vi "ADIS16448 IMU Example.vi"() -> ()   [LabVIEW 2019]
uses:
  <vilib>/Utility/RT CPU Load.ctl
  ADIS16448Lib/Typedef/ADIS16448 Hardware Configuration.ctl
  <vilib>/Rock Robotics/WPI/SPI/WPI_SPIMode.ctl
  <vilib>/Rock Robotics/SystemInterfaces/DIO/FPGA_DIOChannel.ctl
  <vilib>/Rock Robotics/SystemInterfaces/spilib/spi_bus.ctl
  <vilib>/NI_Real-Time Target Support.lvlib
panel:
  in  "Initial Calibration Time (sec)":i32=5
  in  "Hardware Config":T1={"SPI Clock Rate (Hz)"=1000000.0, "IMU SPI Mode (3)"=enum."Mode 3 (Clk Idle High,Sample on Trailing)", "IMU Reset Pin"=enum."DIO MXP 8", "IMU SPI Bus"=enum."SPI MXP", "IMU Data Ready Pin"=enum."DIO MXP 0", "Stall Config"={"Pow2BytesPerRead"=1, "StallTicks"=1000, "CsToSclkTicks"=5}, "IMU Status LED Pin"=enum."DIO MXP 9"}
  in  "Recalibrate?":bool
  in  "Reset?":bool
  out "Integrated Gyro Angle":T5(graph)
  out "Calibrated?":bool
  out "Ready?":bool
  out "CPU loads":T6[](array[typedef]) {"ISR (%)" format="%#.2f"; "Idle (%)" format="%#.2f"; "Background (%)" format="%#.2f"; "Normal (%)" format="%#.2f"; "Above Normal (%)" format="%#.2f"; "High (%)" format="%#.2g"; "Timed Structures (%)" format="%#.2g"; "Time Critical (%)" format="%#.2g"; "Total (%)" format="%#.2g"}
  in  "stop":bool
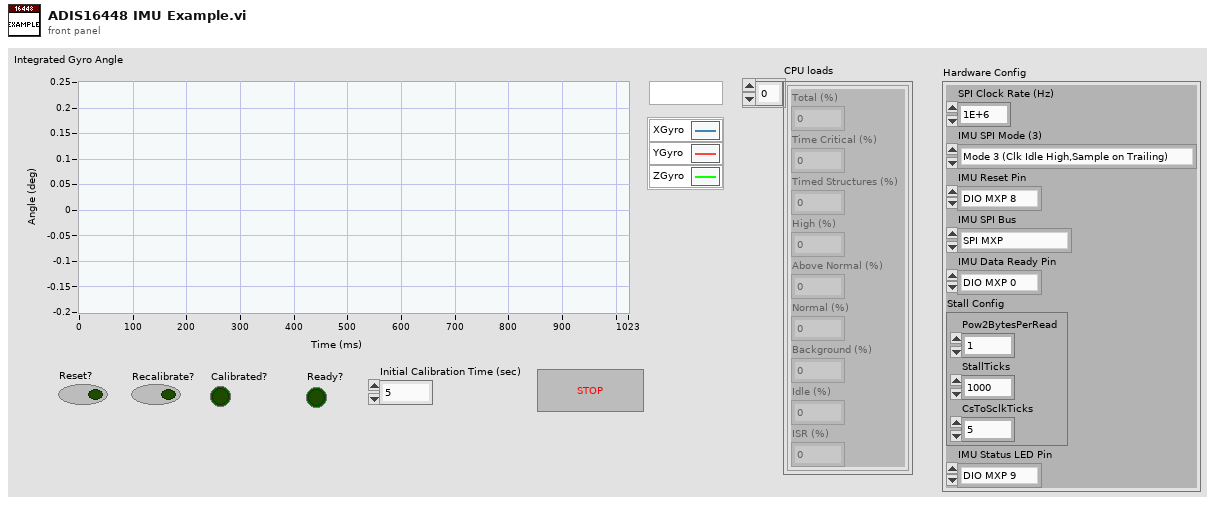
[diagram p1: front panel]
types:
  T1 = typedef "ADIS16448 Hardware Configuration.ctl" = cluster{"SPI Clock Rate (Hz)":dbl, "IMU SPI Mode (3)":T2, "IMU Reset Pin":T3, "IMU SPI Bus":T4, "IMU Data Ready Pin":T3, "Stall Config":cluster{"Pow2BytesPerRead":u8, "StallTicks":u16, "CsToSclkTicks":u8}, "IMU Status LED Pin":T3}
  T2 = typedef "WPI_SPIMode.ctl" = enum16{"Mode 0 (Clk Idle Low,Sample on Leading)", "Mode 1 (Clk Idle Low,Sample on Trailing)", "Mode 2 (Clk Idle High,Sample on Leading)", "Mode 3 (Clk Idle High,Sample on Trailing)"}
  T3 = typedef "FPGA_DIOChannel.ctl" = enum8{"DIO 0", "DIO 1", "DIO 2", "DIO 3", "DIO 4", "DIO 5", "DIO 6", "DIO 7", "DIO 8", "DIO 9", "DIO MXP 0", "DIO MXP 1", "DIO MXP 2", "DIO MXP 3", "DIO MXP 4", "DIO MXP 5", "DIO MXP 6", "DIO MXP 7", "DIO MXP 8", "DIO MXP 9", "DIO MXP 10", "DIO MXP 11", "DIO MXP 12", "DIO MXP 13", "DIO MXP 14", "DIO MXP 15", "SPI Port CS1", "SPI Port CS2", "SPI Port CS3", "SPI Port MISO", "SPI Port MOSI", "Invalid"}
  T4 = typedef "spi_bus.ctl" = enum16{"SPI On-Board, CS0", "SPI On-Board, CS1", "SPI On-Board, CS2", "SPI On-Board, CS3", "SPI MXP", "Invalid"}
  T5 = cluster{"XAngle":dbl, "YAngle":dbl, "ZAngle":dbl}
  T6 = typedef "NI_Real-Time Target Support.lvlib/RT CPU Load.ctl" = cluster{"Total (%)":dbl, "Time Critical (%)":dbl, "Timed Structures (%)":dbl, "High (%)":dbl, "Above Normal (%)":dbl, "Normal (%)":dbl, "Background (%)":dbl, "Idle (%)":dbl, "ISR (%)":dbl}
  T7 = typedef "ADIS16448 Device Reference.ctl" = cluster{"DevStatus":errorcluster, "Hardware Config":T1, "Calibration Complete":refnum<notifier>, "Status FIFO":refnum<k33>, "Last Value Reference":refnum<data-value>, "Sychronous Process VI":T8, "Cmd FIFO":refnum<k33>, "Source":T9, "Data FIFO":refnum<k33>, "IMU Status LED Pin":T3, "Calibration Time":i32}
  T8 = typedef "ADIS16448 Process.ctl" = refnum<vi>
  T9 = typedef "FPGA_CounterEncoderSourceConvertionLVSourceType.ctl" = cluster{"DevStatus":errorcluster, "AnalogTriggerMode?":bool, "DigitalMode":cluster{"DIO Channel":T10}, "AnalogTriggerMode":cluster{"AnalogTriggerIndex":T11, "OutputType":T12}}
  T10 = typedef "FPGA_DIODigitalSourceChannel.ctl" = enum8{"DIO 0", "DIO 1", "DIO 2", "DIO 3", "DIO 4", "DIO 5", "DIO 6", "DIO 7", "DIO 8", "DIO 9", "DIO MXP 0", "DIO MXP 1", "DIO MXP 2", "DIO MXP 3", "DIO MXP 4", "DIO MXP 5", "DIO MXP 6", "DIO MXP 7", "DIO MXP 8", "DIO MXP 9", "DIO MXP 10", "DIO MXP 11", "DIO MXP 12", "DIO MXP 13", "DIO MXP 14", "DIO MXP 15", "SPI Port CS1", "SPI Port CS2", "SPI Port CS3", "SPI Port MISO", "SPI Port MOSI", "Disabled"}
  T11 = typedef "FPGA_AnalogTriggerIndex.ctl" = enum8{"Trig 0", "Trig 1", "Trig 2", "Trig 3", "Trig 4", "Trig 5", "Trig 6", "Trig 7", "Invalid"}
  T12 = typedef "FPGA_AnalogTriggerOutType.ctl" = enum16{"InWindow", "TriggerState", "Rising", "Falling"}
  T13 = typedef "ADIS16448 Status.ctl" = cluster{"Calibrated?":bool}
  T14 = typedef "ADIS16448 Data.ctl" = cluster{"XAngle":dbl, "YAngle":dbl, "ZAngle":dbl}
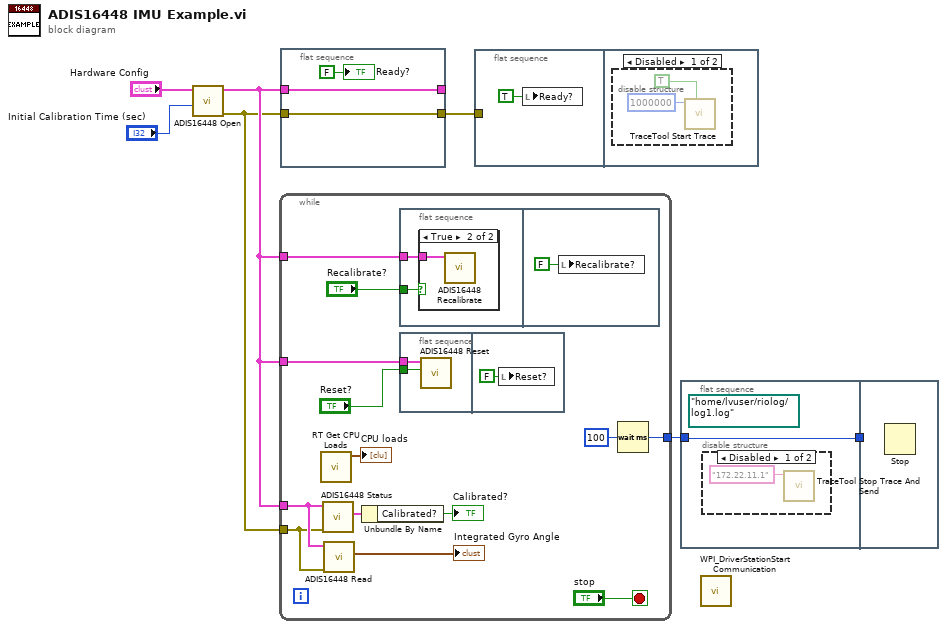
[diagram p0: block diagram]
diagram:
  n1 = call "ADIS16448 Open.vi"("Initial Calibration Time (sec)"="Initial Calibration Time (sec)", "Hardware Config"="Hardware Config") -> ("error out"=w3:errorcluster, "ADIS16448DevRef"=w4:T7)  [unwired: 8 in]
  n2 = while {
    tunnel: [w17] -> w7
    tunnel: w4 -> [w14]
    tunnel: w3 -> [w13]
    tunnel: w4 -> [w11]
    tunnel: w4 -> [w9]
    stop <- "stop" stop-if-true
    n3 = call <vilib>:"RT Get CPU Loads.vi"() -> ("CPU loads"=→"CPU loads":T6[])  [unwired: 10 in, 1 out]
    n4 = call "ADIS16448 Status.vi"("error in (no error)"=w13, "ADIS16448DevRef"=w14) -> ("ADIS16448 Status"=w15:T13)  [unwired: 7 in, 2 out]
    n5 = call "ADIS16448 Read.vi"("error in (no error)"=w13, "ADIS16448DevRef"=w14) -> ("ADIS16448 Value"=→"Integrated Gyro Angle":T14)  [unwired: 6 in, 3 out]
    n6 = Unbundle By Name(w15) -> ("Calibrated?"=→"Calibrated?":bool)
    n7 = flat-sequence {
      tunnel: w9 -> [w22]
      tunnel: "Recalibrate?" -> [w21]
      frame #0 {
        n8 = case shown="True" w21 {
          tunnel: w22 -> [_ w23]
          frame False {
          }
          frame True {
            n9 = call "ADIS16448 Recalibrate.vi"("ADIS16448DevRef in"=w23) -> ()  [unwired: 9 in, 2 out]
          }
        }
      }
      frame #1 {
        n10 = local write "Recalibrate?"(FALSE ("Recalibrate?")) -> ()
      }
    }
    n11 = flat-sequence {
      tunnel: "Reset?" -> [w26]
      tunnel: w11 -> [w25]
      frame #0 {
        n12 = call "ADIS16448 Reset.vi"("Reset?"=w26, "ADIS16448DevRef"=w25) -> ()  [unwired: 8 in, 2 out]
      }
      frame #1 {
        n13 = local write "Reset?"(FALSE ("Reset?")) -> ()
      }
    }
    n14 = Wait (ms)(milliseconds to wait=u32 100) -> (millisecond timer value=w17:u32)
  }
  n15 = flat-sequence {
    tunnel: w4 -> [w29]
    tunnel: [w29] -> _
    tunnel: w3 -> [w28]
    tunnel: [w28] -> w6
    frame #0 {
      "Ready?" <- FALSE ("Ready?")
    }
  }
  n16 = flat-sequence {
    tunnel: w6 -> [_]
    frame #0 {
      n17 = local write "Ready?"(TRUE ("Ready?")) -> ()
    }
    frame #1 {
      n18 = disable-structure shown="Disabled" {
        frame Disabled {
          n19 = call <vilib>:"TraceTool Start Trace.vi"("Detailed Tracing? (F)"=TRUE, "Buffer Size (250000 bytes)"=1000000) -> ()  [unwired: 8 in, 2 out]
        }
        frame Enabled {
        }
      }
    }
  }
  n20 = flat-sequence {
    tunnel: w7 -> [w34]
    tunnel: [w34] -> w5
    tunnel: w5 -> [_]
    frame #0 {
      (unwired) path "/home/lvuser/riolog/log1.log" ("Path to Trace Log")
      n21 = disable-structure shown="Disabled" {
        frame Disabled {
          n22 = call <vilib>:"TraceTool Stop Trace And Send.vi"("Trace Host Network Address"="172.22.11.1") -> ()  [unwired: 10 in, 1 out]
        }
        frame Enabled {
        }
      }
    }
    frame #1 {
      n23 = Stop() -> ()  [unwired: 1 in]
    }
  }
  n24 = call <vilib>:"WPI_DriverStationStart Communication.vi"() -> ()  [unwired: 12 in]
